vi "Set Overtemp.vi"(6 "parseError? T:Yes":bool=TRUE, 8 "error in (no error)":errorcluster, 10 "Overtemp (50.00°C)":dbl=50.0, 11 "VISA resource name":refnum<visa-resource-name>) -> (0 "error out":errorcluster, 3 "VISA resource name out":refnum<visa-resource-name>)   [LabVIEW 2021, in "JULABO DeviceDriver.lvlib"]
doc: "This VI adjusts the higher temperature limit. If for a sensitive temperature application task adherence to a working temperature value >Setpoint< is to be supervised, then set high and low temperature warning values. In case the internal bath temperature exceeds the specified limits, the instrument will show a warning message or will switch to alarm state depending on the settings in the according menu.\n\nNote:\nThe limits reaction is not adjustable via this driver. Please adjust the reaction in the according menu."
uses:
  JULABO DeviceDriver.lvlib
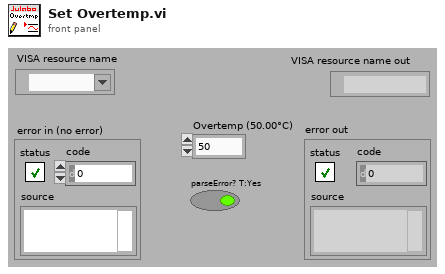
[diagram p1: front panel]
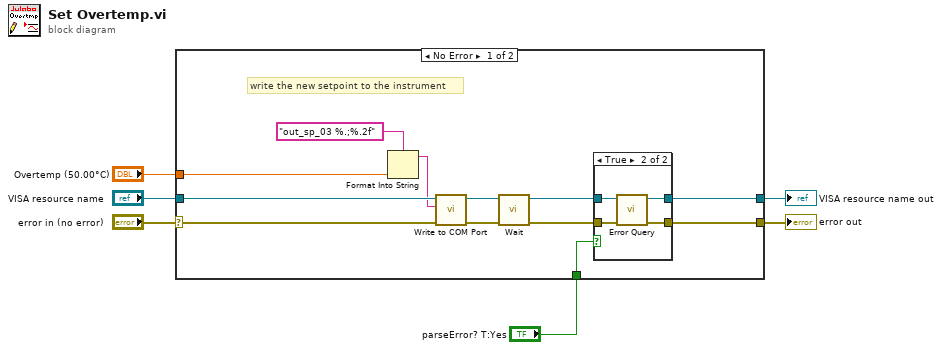
[diagram p0: block diagram]
diagram:
  n1 = case shown="No Error" "error in (no error)" {
    selector: "error in (no error)" -> [w17 w25]
    tunnel: "VISA resource name" -> [w18 w26]
    tunnel: [w15 w25] -> w5
    tunnel: [w14 w26] -> w4
    tunnel: "Overtemp (50.00°C)" -> [w16 _]
    tunnel: "parseError? T:Yes" -> [w13 _]
    frame No Error {
      # "write the new setpoint to the instrument"
      n2 = Format Into String(format string="out_sp_03 %.;%.2f", w16) -> (resulting string=w7:string)  [unwired: 2 in, 1 out]
      n3 = call "Write to COM Port.vi"("error in"=w17, "Command (input)"=w7, "VISA resource name in"=w18) -> ("error out"=w11:errorcluster, "VISA resource name out"=w12:refnum<visa-resource-name>)  [unwired: 7 in]
      n4 = call "Wait.vi"("error in"=w11, "VISA resource name in"=w12) -> ("error out"=w9:errorcluster, "VISA resource name out"=w10:refnum<visa-resource-name>)  [unwired: 4 in]
      n5 = case shown="True" w13 {
        tunnel: w10 -> [w20 w24]
        tunnel: w9 -> [w19 w23]
        tunnel: [w20 w22] -> w14
        tunnel: [w19 w21] -> w15
        frame False {
        }
        frame True {
          n6 = call "Error Query.vi"("error in (no error)"=w23, "VISA resource name"=w24) -> ("error out"=w21:errorcluster, "VISA resource name out"=w22:refnum<visa-resource-name>)  [unwired: 6 in, 2 out]
        }
      }
    }
    frame Error {
    }
  }
  "error out" <- w5
  "VISA resource name out" <- w4
